vi "Test All.vi"(8 "error in (no error)":errorcluster) -> (0 "error out":errorcluster)   [LabVIEW 2013]
doc: "This example demonstrates how to test a LabVIEW class library functionality using a simple dictionary class as an example."
uses:
  classes/Test/Test.lvclass
panel:
  # "See block diagram"
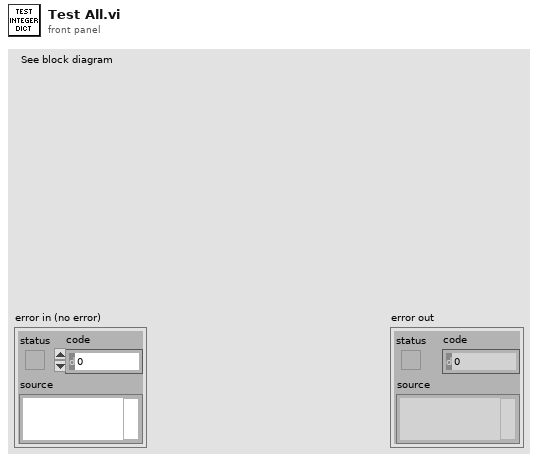
[diagram p1: front panel]
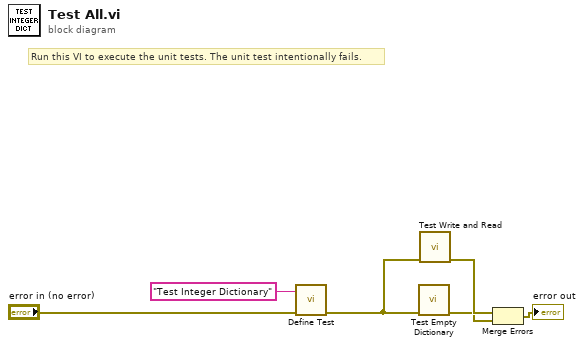
[diagram p0: block diagram]
diagram:
  # "Run this VI to execute the unit tests. The unit test intentionally fails."
  n1 = call "Define Test.vi"("error in (no error)"="error in (no error)", "Label (VI Title)"="Test Integer Dictionary") -> ("error out"=w3:errorcluster)  [unwired: 8 in, 1 out]
  n2 = call "Test Empty Dictionary.vi"("error in (no error)"=w3) -> ("error out"=w1:errorcluster)  [unwired: 10 in]
  n3 = call "Test Write and Read.vi"("error in (no error)"=w3) -> ("error out"=w2:errorcluster)  [unwired: 10 in]
  n4 = Merge Errors(w2, w1) -> (→"error out":errorcluster)
